vi "BlobLineMerger.vi"() -> ()   [LabVIEW 2011]
uses:
  <vilib>/Analysis/NI_AAL_Geometry.lvlib
  <vilib>/Analysis/geometry.llb/Point in Polygon (Scalar).vi
panel:
  out "BlobLineData":T1
  in  "Lines":T2(array[cluster])
  in  "Blob Array":T3(array[cluster])
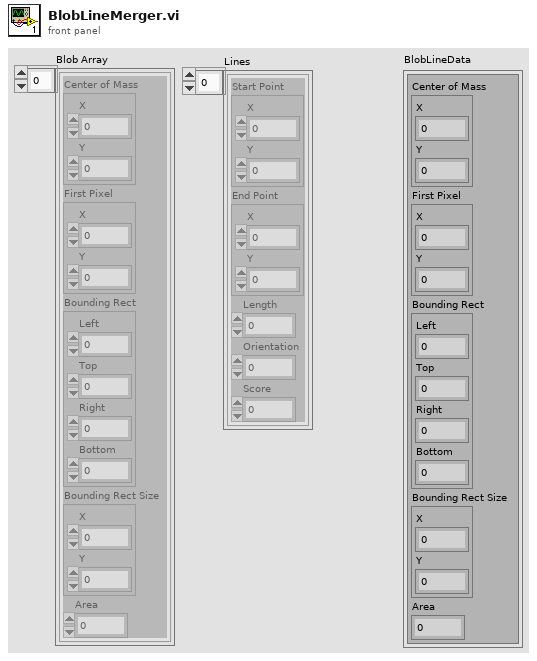
[diagram p1: front panel]
types:
  T1 = cluster{"Blob":cluster{"Center of Mass":cluster{"X":dbl, "Y":dbl}, "First Pixel":cluster{"X":dbl, "Y":dbl}, "Bounding Rect":cluster{"Left":dbl, "Top":dbl, "Right":dbl, "Bottom":dbl}, "Bounding Rect Size":cluster{"X":dbl, "Y":dbl}, "Area":dbl}}
  T2 = cluster{"Start Point":cluster{"X":sgl, "Y":sgl}, "End Point":cluster{"X":sgl, "Y":sgl}, "Length":dbl, "Orientation":dbl, "Score":dbl}[]
  T3 = cluster{"Center of Mass":cluster{"X":dbl, "Y":dbl}, "First Pixel":cluster{"X":dbl, "Y":dbl}, "Bounding Rect":cluster{"Left":dbl, "Top":dbl, "Right":dbl, "Bottom":dbl}, "Bounding Rect Size":cluster{"X":dbl, "Y":dbl}, "Area":dbl}[]
  T4 = cluster{"Left":dbl, "Top":dbl, "Right":dbl, "Bottom":dbl}
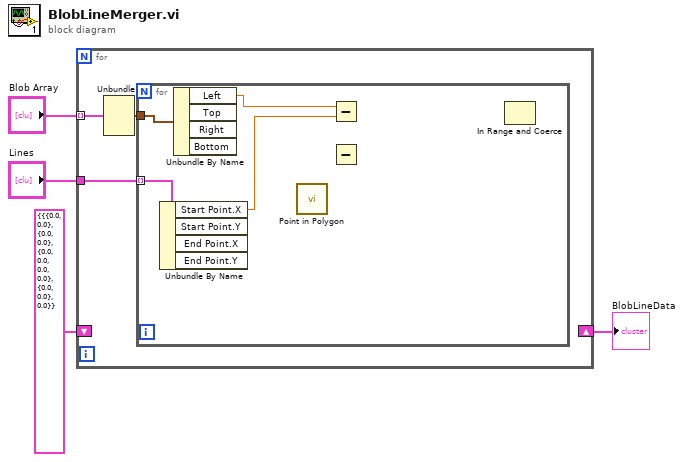
[diagram p0: block diagram]
diagram:
  n1 = for {
    tunnel: "Blob Array" -> [w6] mode=indexing
    tunnel: "Lines" -> [w7]
    shift-right: [_] -> w1
    shift-left: T1 {"Blob"={"Center of Mass"={"X"=0.0, "Y"=0.0}, "First Pixel"={"X"=0.0, "Y"=0.0}, "Bounding Rect"={"Left"=0.0, "Top"=0.0, "Right"=0.0, "Bottom"=0.0}, "Bounding Rect Size"={"X"=0.0, "Y"=0.0}, "Area"=0.0}} ("BlobLineData") -> [_]
    n2 = Unbundle(w6) -> ("Bounding Rect"=w5:T4)  [unwired: 4 out]
    n3 = for {
      tunnel: w7 -> [w11] mode=indexing
      tunnel: w5 -> [w10]
      n4 = Unbundle By Name(w11) -> ("Start Point.X"=w8:sgl)  [unwired: 3 out]
      n5 = Unbundle By Name(w10) -> ("Left"=w9:dbl)  [unwired: 3 out]
      n6 = call-poly <vilib>:"Point in Polygon.vi"() -> ()  [unwired: 10 in, 2 out]
      n7 = Subtract(x=w9, y=w8) -> ()  [unwired: 1 out]
      n8 = Subtract() -> ()  [unwired: 2 in, 1 out]
      n9 = In Range and Coerce() -> ()  [unwired: 3 in, 2 out]
    }
  }
  "BlobLineData" <- w1
